vi "List End.vi"(6 "Output State":bool, 8 "error in":errorcluster, 11 "VISA resource name":refnum<visa-resource-name>) -> (0 "error out":errorcluster, 3 "VISA resource name":refnum<visa-resource-name>)   [LabVIEW 2022 SP3]
uses:
  <instrlib>/BK Precision 911X Series/BK Precision 911X Series.lvlib
panel:
  out "Stop":i32
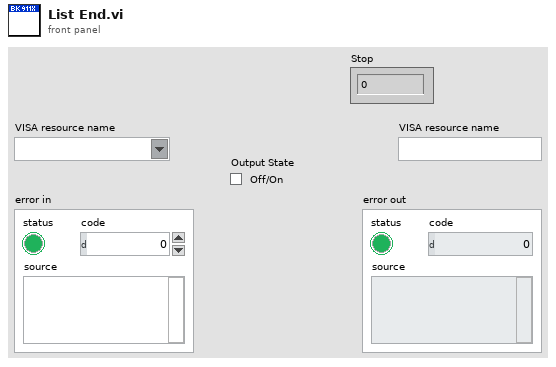
[diagram p1: front panel]
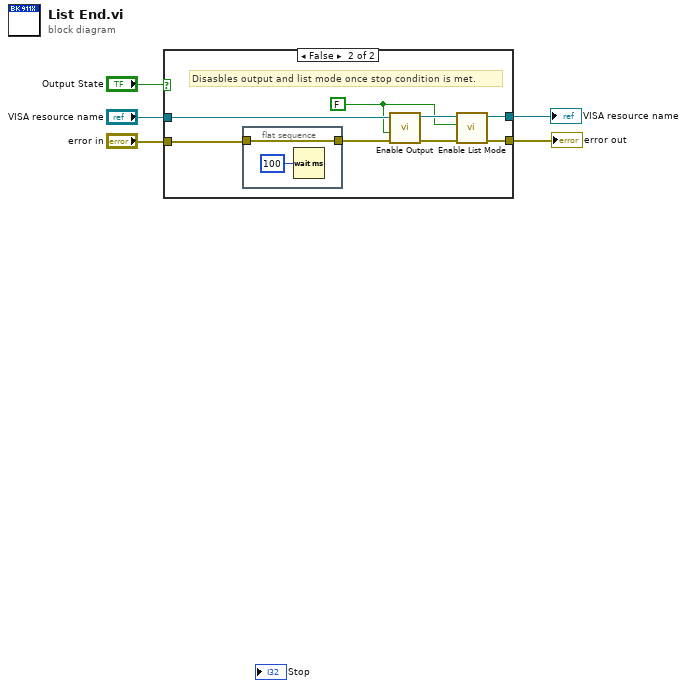
[diagram p0: block diagram]
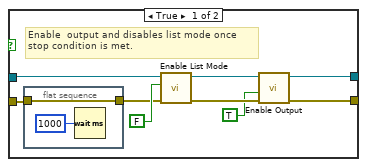
[diagram p2: hidden frame]
diagram:
  n1 = case shown="False" "Output State" {
    tunnel: [w10 w21] -> w5
    tunnel: [w9 w20] -> w4
    tunnel: "error in" -> [w14 w19]
    tunnel: "VISA resource name" -> [w7 w18]
    frame True {
      # "Enable  output and disables list mode once \nstop condition is met."
      n2 = flat-sequence {
        tunnel: w14 -> [w15]
        tunnel: [w15] -> w12
        frame #0 {
          n3 = Wait (ms)(milliseconds to wait=u32 1000) -> ()  [unwired: 1 out]
        }
      }
      n4 = call <instrlib>:"Enable List Mode.vi"("error in (no error)"=w12, "Enable List Mode (F: False)"=FALSE, "VISA resource name"=w7) -> ("error out"=w11:errorcluster, "VISA resource name out"=w8:refnum<visa-resource-name>)  [unwired: 7 in]
      n5 = call <instrlib>:"Enable Output.vi"("error in (no error)"=w11, "Enable Output (F: False)"=TRUE, "VISA resource name"=w8) -> ("error out"=w10:errorcluster, "VISA resource name out"=w9:refnum<visa-resource-name>)  [unwired: 7 in]
    }
    frame False {
      w17 = FALSE ("Enable Output (F: False)")
      # "Disasbles output and list mode once stop condition is met."
      n6 = flat-sequence {
        tunnel: w19 -> [w25]
        tunnel: [w25] -> w24
        frame #0 {
          n7 = Wait (ms)(milliseconds to wait=u32 100) -> ()  [unwired: 1 out]
        }
      }
      n8 = call <instrlib>:"Enable Output.vi"("error in (no error)"=w24, "Enable Output (F: False)"=w17, "VISA resource name"=w18) -> ("error out"=w23:errorcluster, "VISA resource name out"=w22:refnum<visa-resource-name>)  [unwired: 7 in]
      n9 = call <instrlib>:"Enable List Mode.vi"("error in (no error)"=w23, "Enable List Mode (F: False)"=w17, "VISA resource name"=w22) -> ("error out"=w21:errorcluster, "VISA resource name out"=w20:refnum<visa-resource-name>)  [unwired: 7 in]
    }
  }
  "VISA resource name" <- w4
  "error out" <- w5
